vi "subVI_tf_a_espacio_de_estado.vi"(4 "Retardo":dbl format="%.2f segundos", 5 "Denominador":dbl[](array[numeric]), 6 "Numerador":dbl[](array[numeric])) -> (0 "C":dbl[](array[numeric]), 2 "B":dbl[](array[numeric]), 3 "A":T1)   [LabVIEW 2018]
uses:
  <vilib>/Analysis/Matrix/NI_Matrix.lvlib
  <vilib>/Analysis/NI_AALBase.lvlib
  <vilib>/Analysis/Matrix/Numeric/Conversions/Array To Matrix - RA.vi
  <vilib>/Analysis/NI_AALPro.lvlib
  <vilib>/Analysis/polynomials.llb/Multiply Polynomials (DBL).vi
  <vilib>/Analysis/Matrix/Numeric/Conversions/Array To Matrix - RA2.vi
  <vilib>/Analysis/Matrix/Numeric/Multiply/Multiply - RM,R.vi
  <vilib>/Analysis/7linalg.llb/Real Matrix Power.vi
  <vilib>/Analysis/Matrix/Datatypes/RealMatrix.ctl
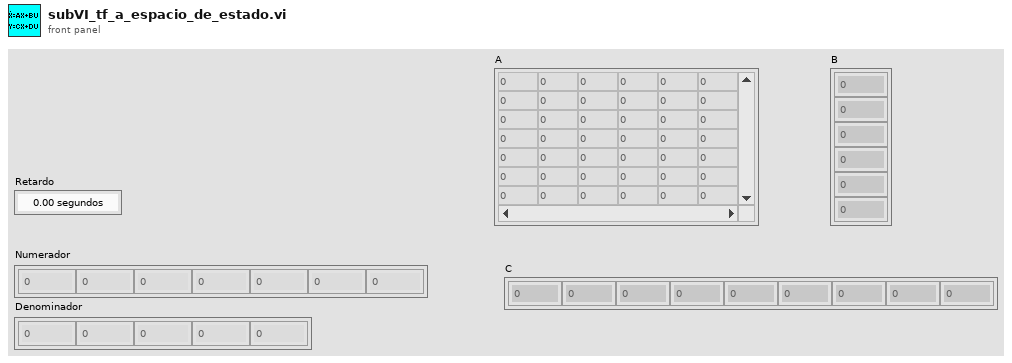
[diagram p1: front panel]
types:
  T1 = typedef "NI_Matrix.lvlib/RealMatrix.ctl" = dbl[][]
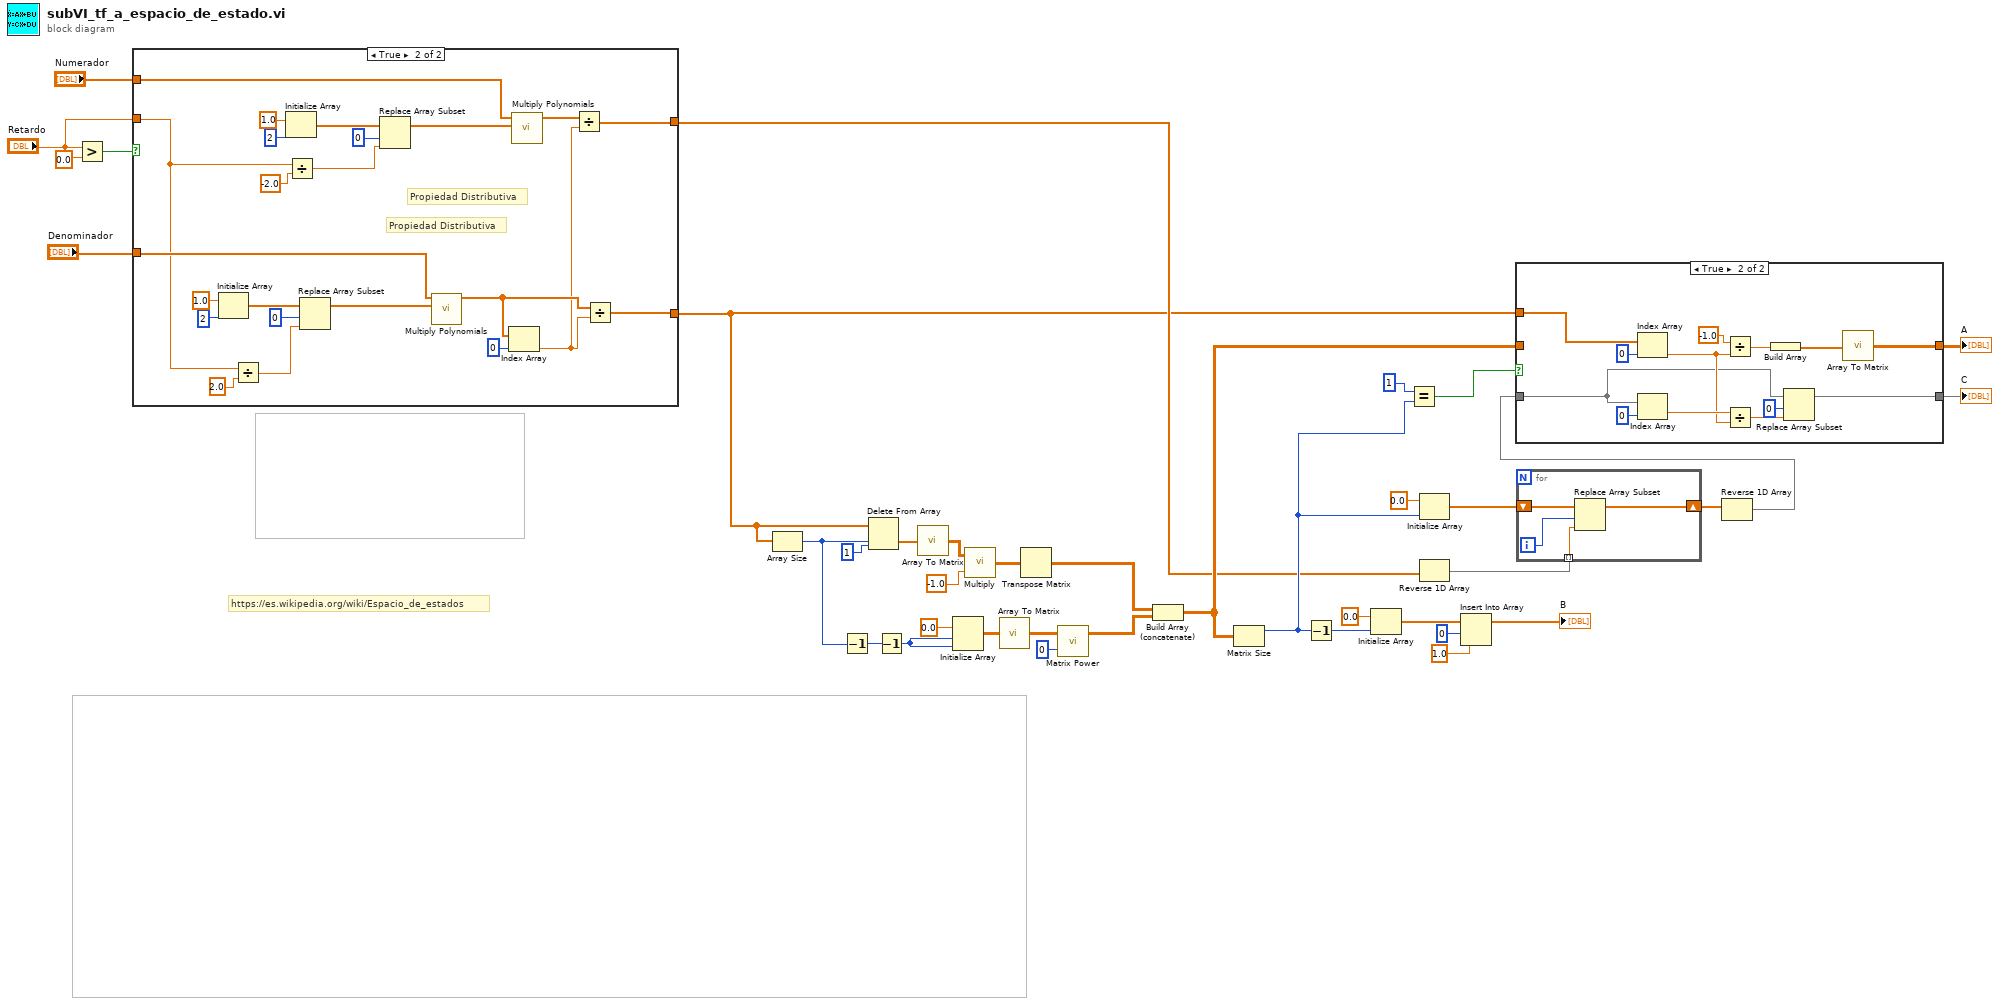
[diagram p0: block diagram]
diagram:
  # "https://es.wikipedia.org/wiki/Espacio_de_estados"
  n1 = Greater?(x="Retardo", y=0.0) -> (0:w8:bool)
  n2 = case shown="True" w8 {
    tunnel: "Retardo" -> [_ w44]
    tunnel: "Numerador" -> [w40 w59]
    tunnel: [w40 w48] -> w5
    tunnel: "Denominador" -> [w39 w54]
    tunnel: [w39 w51] -> w3
    frame False {
    }
    frame True {
      # "Propiedad Distributiva"
      # "Propiedad Distributiva"
      n3 = Initialize Array "Initialize Array"(1.0 ("element"), 2 ("dimension size")) -> (w55:dbl[])
      n4 = Divide(x=w44, y=2.0) -> (x/y=w42:dbl)
      n5 = Initialize Array "Initialize Array"(1.0 ("element"), 2 ("dimension size")) -> (w63:dbl[])
      n6 = Divide(x=w44, y=-2.0) -> (x/y=w46:dbl)
      n7 = Replace Array Subset "Replace Array Subset"(array=w55, new element=w42, index=0) -> (w58:dbl[])
      n8 = Replace Array Subset "Replace Array Subset"(array=w63, new element=w46, index=0) -> (w60:dbl[])
      n9 = call-poly <vilib>:"Multiply Polynomials.vi"("Q(x)"=w58, "P(x)"=w54) -> ("P(x)*Q(x)"=w52:dbl[])  [unwired: 8 in, 1 out]
      n10 = Index Array "Index Array"(array=w52, index=0) -> (element=w49:dbl)
      n11 = call-poly <vilib>:"Multiply Polynomials.vi"("Q(x)"=w60, "P(x)"=w59) -> ("P(x)*Q(x)"=w50:dbl[])  [unwired: 8 in, 1 out]
      n12 = Divide(x=w50, y=w49) -> (x/y=w48:dbl[])
      n13 = Divide(x=w52, y=w49) -> (x/y=w51:dbl[])
    }
  }
  n14 = Array Size(array=w3) -> (size(s)=w29:i32)
  n15 = Decrement(x=w29) -> (x-1=w28:i32)
  n16 = Delete From Array "Delete From Array"(array=w3, length=w29, index=1) -> (deleted portion=w37:dbl[])  [unwired: 1 out]
  n17 = Decrement(x=w28) -> (x-1=w32:i32)
  n18 = call-poly <vilib>:"Array To Matrix.vi"("Real 1D Array"=w37) -> ("Real Matrix (Column Vector)"=w36:T1)
  n19 = Initialize Array "Initialize Array"(0.0, w32, w32) -> (w31:dbl[][])
  n20 = call-poly <vilib>:"Multiply.vi"("Real Scalar c"=-1.0, "Real Matrix A"=w36) -> ("A * c"=w27:T1)
  n21 = call-poly <vilib>:"Array To Matrix.vi"("Real 2D Array"=w31) -> ("Real Matrix"=w30:T1)
  n22 = Transpose Matrix(1:w27) -> (0:w26:T1)
  n23 = call-poly <vilib>:"Matrix Power.vi"("n"=0, "Input Matrix"=w30) -> ("Matrix Power"=w25:T1)  [unwired: 1 out]
  n24 = Build Array (concatenate)(w26, w25) -> (w13:T1)
  n25 = Matrix Size(0:w13) -> (1:w10:i32)  [unwired: 1 out]
  n26 = Decrement(x=w10) -> (x-1=w20:i32)
  n27 = Initialize Array "Initialize Array"(0.0, w20) -> (w19:dbl[])
  n28 = Equal?(x=1, y=w10) -> (x = y?=w12:bool)
  n29 = Initialize Array "Initialize Array"(0.0, w10) -> (w17:dbl[])
  n30 = Reverse 1D Array(array=w5) -> (reversed array=w15:dbl[])
  n31 = Insert Into Array "Insert Into Array"(array=w19, index=0, new element=1.0 ("new element/subarray")) -> (→"B":dbl[])
  n32 = for {
    shift-right: [w65] -> w16
    shift-left: w17 -> [w67]
    tunnel: w15 -> [w64] mode=indexing
    i -> [w66]
    n33 = Replace Array Subset "Replace Array Subset"(array=w67, new element=w64, index=w66) -> (w65:dbl[])
  }
  n34 = Reverse 1D Array(array=w16) -> (reversed array=w1:dbl[])
  n35 = case shown="True" w12 {
    tunnel: w13 -> [w69 _]
    tunnel: [w69 w80] -> w11
    tunnel: w3 -> [_ w77]
    tunnel: w1 -> [w68 w73]
    tunnel: [w68 w70] -> w2
    frame False {
    }
    frame True {
      n36 = Index Array "Index Array"(array=w77, index=0) -> (element=w74:dbl)
      n37 = Index Array "Index Array"(array=w73, index=0) -> (element=w75:dbl)
      n38 = Divide(x=-1.0, y=w74) -> (x/y=w78:dbl)
      n39 = Divide(x=w75, y=w74) -> (x/y=w71:dbl)
      n40 = Build Array "Build Array"(w78) -> (w81:dbl[])
      n41 = Replace Array Subset "Replace Array Subset"(array=w73, new element=w71, index=0) -> (w70:dbl[])
      n42 = call-poly <vilib>:"Array To Matrix.vi"("Real 1D Array"=w81) -> ("Real Matrix (Column Vector)"=w80:T1)
    }
  }
  "A" <- w11
  "C" <- w2
